vi "Mallet Move V2.vi"(8 "Forward":u8, 9 "Reverse":u8) -> ()   [LabVIEW 2013]
doc: "An example that reads a user selectable analog input pin on the Arduino."
uses:
  <vilib>/LabVIEW Interface for Arduino/Type Defs/Pin Mode.ctl
  <vilib>/LabVIEW Interface for Arduino/LabVIEW Interface for Arduino.lvlib
panel:
  in  "Time2":dbl=0.95 format="%#_13g"
  in  "Time1":dbl=0.95 format="%#_13g"
  in  "Forward 2":u8
  in  "Reverse 2":u8
  in  "stop 2":bool
  in  "stop":bool
  in  "PWM1 Pin":u8
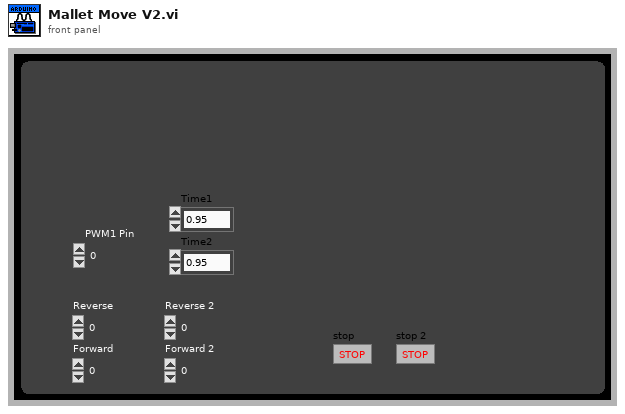
[diagram p1: front panel]
types:
  T1 = typedef "LabVIEW Interface for Arduino.lvlib/Pin Mode.ctl" = enum8{"Input", "Output"}
  T2 = typedef "LabVIEW Interface for Arduino.lvlib/Arduino Resource.ctl" = cluster{"VISA resource":refnum<visa-resource-name>, "Board Type":T3, "Connection Type":enum8{"USB / Serial"}, "Bytes Per Packet (15)":u8}
  T3 = typedef "LabVIEW Interface for Arduino.lvlib/Board Type.ctl" = enum16{"Uno", "Dimuelanove w/Atmega 328", "Mega 2560"}
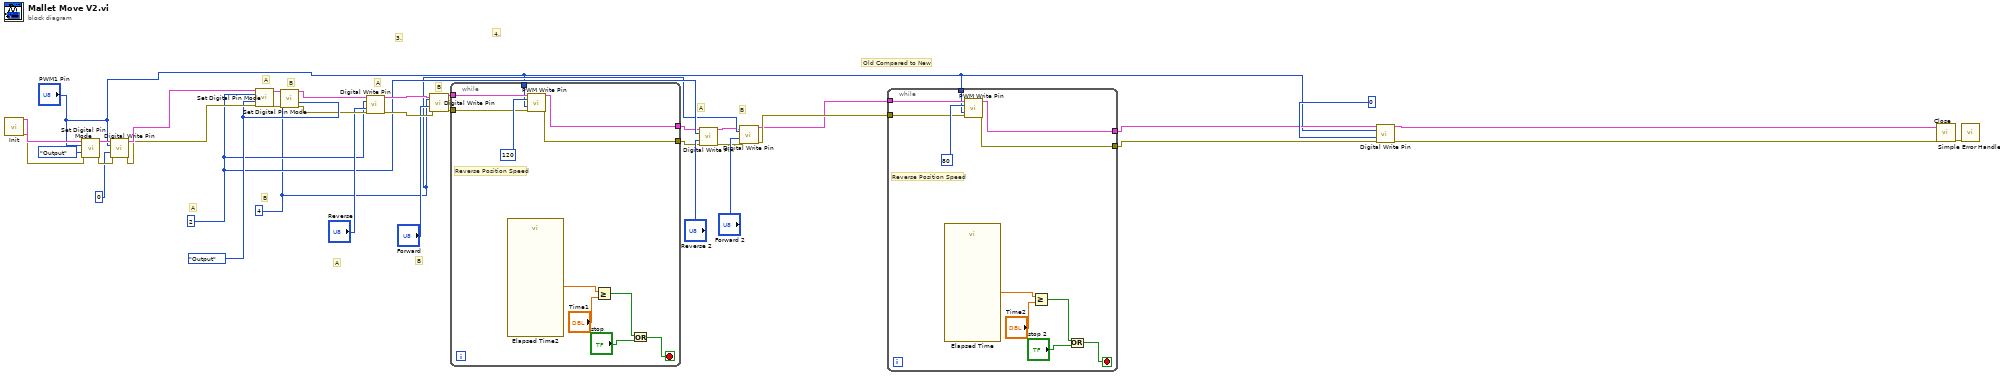
[diagram p0: block diagram]
diagram:
  w10 = u8 4 ("Digital I/O Pin")
  w11 = u8 2 ("Digital I/O Pin")
  w24 = Pin_Mode."Output" ("Pin Mode (Input)")
  # "B"
  # "A"
  # "Old Compared to New"
  # "4."
  # "3."
  # "B"
  # "A"
  # "B"
  # "A"
  # "B"
  # "A"
  # "B"
  # "A"
  n1 = call <vilib>:"Init.vi"() -> ("Arduino Resource"=w28:T2, "error out"=w27:errorcluster)  [unwired: 18 in]
  n2 = call <vilib>:"Set Digital Pin Mode.vi"("Arduino Resource"=w28, "Digital I/O Pin"="PWM1 Pin", "Pin Mode (Input)"=Pin_Mode."Output", "error in"=w27) -> ("Arduino Resource"=w33:T2, "error out"=w32:errorcluster)  [unwired: 10 in]
  n3 = call <vilib>:"Digital Write Pin.vi"("Arduino Resource"=w33, "Digital I/O Pin (0)"="PWM1 Pin", "Value (0)"=u8 0, "error in"=w32) -> ("Arduino Resource"=w30:T2, "error out"=w29:errorcluster)  [unwired: 10 in]
  n4 = call <vilib>:"Set Digital Pin Mode.vi"("Arduino Resource"=w30, "Digital I/O Pin"=w11, "Pin Mode (Input)"=w24, "error in"=w29) -> ("Arduino Resource"=w23:T2, "error out"=w22:errorcluster)  [unwired: 10 in]
  n5 = call <vilib>:"Set Digital Pin Mode.vi"("Arduino Resource"=w23, "Digital I/O Pin"=w10, "Pin Mode (Input)"=w24, "error in"=w22) -> ("Arduino Resource"=w19:T2, "error out"=w18:errorcluster)  [unwired: 10 in]
  n6 = call <vilib>:"Digital Write Pin.vi"("Arduino Resource"=w19, "Digital I/O Pin (0)"=w11, "Value (0)"="Reverse", "error in"=w18) -> ("Arduino Resource"=w21:T2, "error out"=w20:errorcluster)  [unwired: 10 in]
  n7 = call <vilib>:"Digital Write Pin.vi"("Arduino Resource"=w21, "Digital I/O Pin (0)"=w10, "Value (0)"="Forward", "error in"=w20) -> ("Arduino Resource"=w15:T2, "error out"=w14:errorcluster)  [unwired: 10 in]
  n8 = while {
    tunnel: w15 -> [w46]
    tunnel: w14 -> [w45]
    tunnel: "PWM1 Pin" -> [w44]
    tunnel: [w43] -> w9
    tunnel: [w42] -> w7
    stop <- w37 stop-if-true
    # "Reverse Position Speed"
    n9 = call "Elapsed Time2"() -> ("Elapsed Time (s)"=w40:dbl)  [unwired: 12 in, 7 out]
    n10 = call <vilib>:"PWM Write Pin.vi"("Arduino Resource"=w46, "Duty Cycle (0 - 255)"=u8 120, "PWM Pin (3)"=w44, "error in"=w45) -> ("Arduino Resource"=w43:T2, "error out"=w42:errorcluster)  [unwired: 10 in]
    n11 = Greater Or Equal?(x=w40, y="Time1") -> (x >= y?=w39:bool)
    n12 = Or(x=w39, y="stop") -> (x .or. y?=w37:bool)
  }
  n13 = call <vilib>:"Digital Write Pin.vi"("Arduino Resource"=w9, "Digital I/O Pin (0)"=w11, "Value (0)"="Reverse 2", "error in"=w7) -> ("Arduino Resource"=w8:T2, "error out"=w6:errorcluster)  [unwired: 10 in]
  n14 = call <vilib>:"Digital Write Pin.vi"("Arduino Resource"=w8, "Digital I/O Pin (0)"=w10, "Value (0)"="Forward 2", "error in"=w6) -> ("Arduino Resource"=w4:T2, "error out"=w5:errorcluster)  [unwired: 10 in]
  n15 = while {
    tunnel: [w57] -> w3
    tunnel: [w56] -> w2
    tunnel: w5 -> [w50]
    tunnel: w4 -> [w49]
    tunnel: "PWM1 Pin" -> [w48]
    stop <- w51 stop-if-true
    # "Reverse Position Speed"
    n16 = call "Elapsed Time"() -> ("Elapsed Time (s)"=w54:dbl)  [unwired: 12 in, 7 out]
    n17 = call <vilib>:"PWM Write Pin.vi"("Arduino Resource"=w49, "Duty Cycle (0 - 255)"=u8 80, "PWM Pin (3)"=w48, "error in"=w50) -> ("Arduino Resource"=w57:T2, "error out"=w56:errorcluster)  [unwired: 10 in]
    n18 = Greater Or Equal?(x=w54, y="Time2") -> (x >= y?=w53:bool)
    n19 = Or(x=w53, y="stop 2") -> (x .or. y?=w51:bool)
  }
  n20 = call <vilib>:"Digital Write Pin.vi"("Arduino Resource"=w3, "Digital I/O Pin (0)"="PWM1 Pin", "Value (0)"=u8 0, "error in"=w2) -> ("Arduino Resource"=w35:T2, "error out"=w34:errorcluster)  [unwired: 10 in]
  n21 = call <vilib>:"Close.vi"("Arduino Resource"=w35, "error in"=w34) -> ("error out"=w36:errorcluster)  [unwired: 13 in]
  n22 = call <vilib>:"Simple Error Handler.vi"("error in (no error)"=w36) -> ()  [unwired: 4 in, 5 out]
